vi "New User.vi"(8 "error in (no error)":errorcluster, 10 "user info":T1, 11 "[Data] Userinfo Binary in":refnum<class "[Data] Userinfo Binary.lvclass">) -> (0 "error out":errorcluster, 3 "[Data] Userinfo Binary out":refnum<class "[Data] Userinfo Binary.lvclass">)   [LabVIEW 2020, in "[Data] Userinfo Binary.lvclass"]
uses:
  [Data] Userinfo Binary.lvclass
  [Data] Abstruct Userinfo/Control/user info.ctl
  Control/user info.ctl
  [Data] Userinfo Binary.lvclass/[Data] Userinfo Binary.ctl
  [Data] Abstruct Userinfo/[Data] Abstruct Userinfo.lvclass
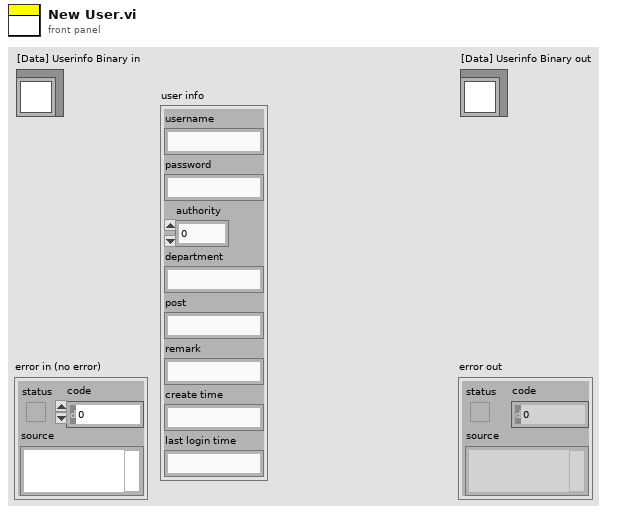
[diagram p1: front panel]
types:
  T1 = typedef "[Data] Abstruct Userinfo.lvclass/user info.ctl" = cluster{"username":string, "password":string, "authority":i8, "department":string, "post":string, "remark":string, "create time":string, "last login time":string}
  T2 = typedef "[Data] Userinfo Binary.lvclass/user info.ctl" = cluster{"password":string, "authority":i8, "department":string, "post":string, "remark":string, "create time":string, "last login time":string}
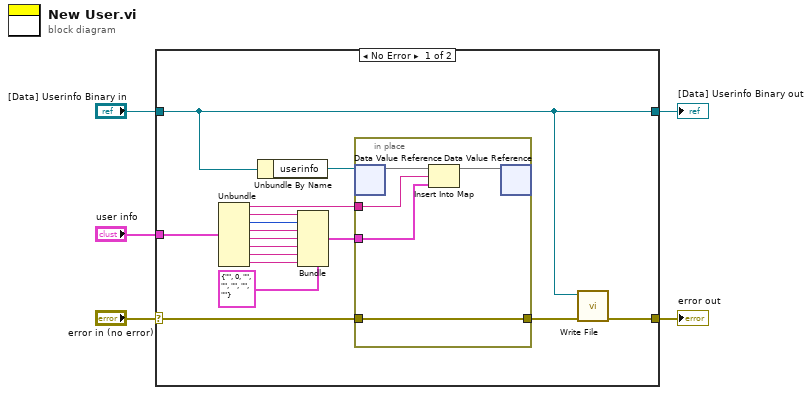
[diagram p0: block diagram]
diagram:
  n1 = case shown="No Error" "error in (no error)" {
    selector: "error in (no error)" -> [w8 w28]
    tunnel: [w6 w28] -> w2
    tunnel: "[Data] Userinfo Binary in" -> [w7 w27]
    tunnel: [w7 w27] -> w4
    tunnel: "user info" -> [w9 _]
    frame No Error {
      n2 = Unbundle(w9) -> ("username"=w11:string, "password"=w14:string, "authority"=w15:i8, "department"=w16:string, "post"=w17:string, "remark"=w18:string, "create time"=w19:string, "last login time"=w20:string)
      n3 = Unbundle By Name(w7) -> ("userinfo"=w13:refnum<data-value>)
      n4 = Bundle(cluster=T2 {"password"="", "authority"=0, "department"="", "post"="", "remark"="", "create time"="", "last login time"=""} ("user info"), "password"=w14, "authority"=w15, "department"=w16, "post"=w17, "remark"=w18, "create time"=w19, "last login time"=w20) -> (w12:T2)
      n5 = in-place {
        in-place-border: w12 -> [w24]
        in-place-border: w11 -> [w25]
        in-place-border: w8 -> [w22]
        in-place-border: [w22] -> w10
        n6 = in-place-dvr #1(w13) -> (w26:map{string, T2})  [unwired: 1 out]
        n7 = Insert Into Map(map in=w26, key=w25, value=w24) -> (map out=w23:map{string, T2})  [unwired: 2 out]
        n8 = in-place-dvr #1(w23) -> ()  [unwired: 2 out]
      }
      n9 = call "Write File.vi"("error in (no error)"=w10, "[Data] Userinfo Binary in"=w7) -> ("error out"=w6:errorcluster)  [unwired: 8 in, 1 out]
    }
    frame Error {
    }
  }
  "error out" <- w2
  "[Data] Userinfo Binary out" <- w4
